vi "Main VI task 2 (copy).vi"() -> ()   [LabVIEW 2024]
panel:
  in  "I_1":dbl
  out "I":dbl
  out "I_sh":dbl
  in  "V":dbl
  out "I_0":dbl
  out "I_rs":dbl
  in  "G":dbl
  out "I_ph":dbl
  in  "T":dbl
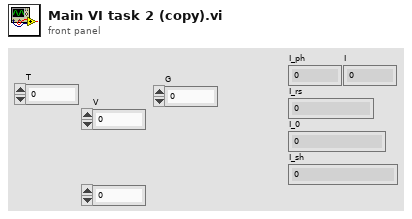
[diagram p1: front panel]
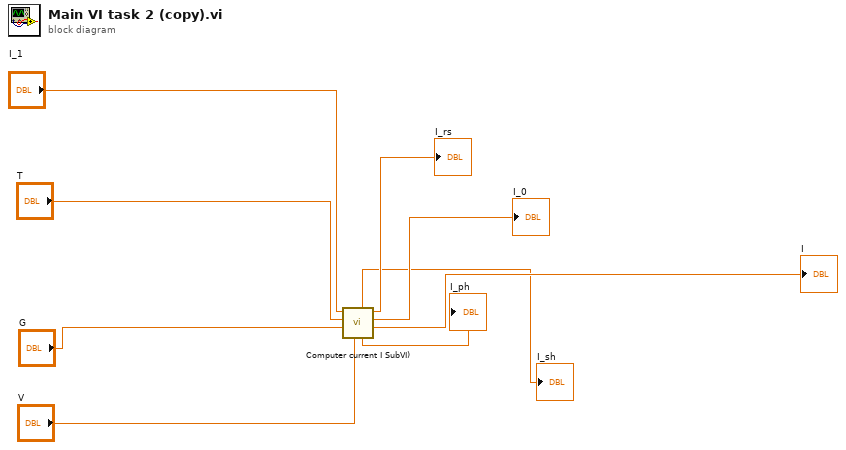
[diagram p0: block diagram]
diagram:
  n1 = call "Computer current I SubVI).vi"("V"="V", "G"="G", "T"="T", "I_1"="I_1") -> ("I"=→"I":dbl, "I_0"=→"I_0":dbl, "I_rs"=→"I_rs":dbl, "I_ph"=→"I_ph":dbl, "I_sh"=→"I_sh":dbl)  [unwired: 3 in]
